vi "Rotation3d_Interpolate.vi"(9 "T":dbl, 10 "EndValue Rotation3d":T1={"Q_quaternion"={"R"=1.0, "V"=[0.0, 0.0, 0.0]}}, 11 "in Rotation3d":T1={"Q_quaternion"={"R"=1.0, "V"=[0.0, 0.0, 0.0]}}) -> (3 "Interpolated Rotation3d":T1={"Q_quaternion"={"R"=1.0, "V"=[0.0, 0.0, 0.0]}})   [LabVIEW 2019, in "Trajectory_Library.lvlib"]
doc: "Interpolates between 2 Rotation3d.\n\nParameters:\n - IN ROTATION3D -- This rotation3d data structure\n - End Value ROTATION3D -- The end rotation3d\n - T -- Interpolation value between 0 and 1.\n\nReturns:\n- Interpolated Rotation3d -- The Rotation3d interpolated betwee the 2 provided interpolations."
uses:
  Trajectory_Library.lvlib
  ROTATION3D.ctl
  QUATERNION.ctl
  Rotation3d_UnaryMinus.vi
  Rotation3d_RotateBy.vi
  Rotation3d_Create_AxisAngle.vi
  Rotation3d_GetQuaterion.vi
  Quaternion_Get_Vect.vi
  Quaternion_Get_W.vi
  Rotation3d_Create_Quaternion.vi
  Quaternion_Inverse.vi
  Quaternion_Times.vi
  Matrix_NormF.vi
  Quaternion_New.vi
  Rotation3d_Create_Default.vi
  Quaternion_Normalize.vi
  <vilib>/Analysis/_algsub.llb/Matrix Norm.vi
  <vilib>/Analysis/_algsub.llb/Real Matrix Norm.vi
  Quaternion_New_Default.vi
  <vilib>/Analysis/Matrix/Numeric/Conversions/Array To Matrix.vi
  <vilib>/Analysis/Matrix/Numeric/Conversions/Array To Matrix - RA.vi
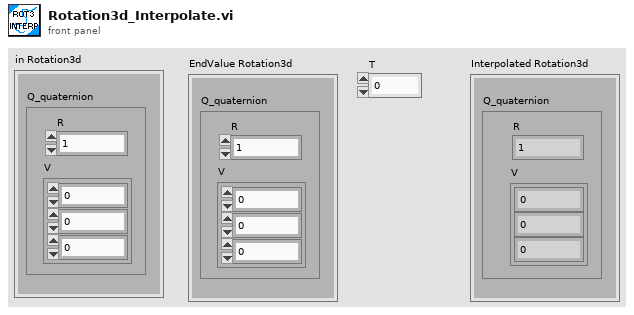
[diagram p1: front panel]
types:
  T1 = typedef "Trajectory_Library.lvlib/ROTATION3D.ctl" = cluster{"Q_quaternion":T2}
  T2 = typedef "Trajectory_Library.lvlib/QUATERNION.ctl" = cluster{"R":dbl, "V":dbl[]}
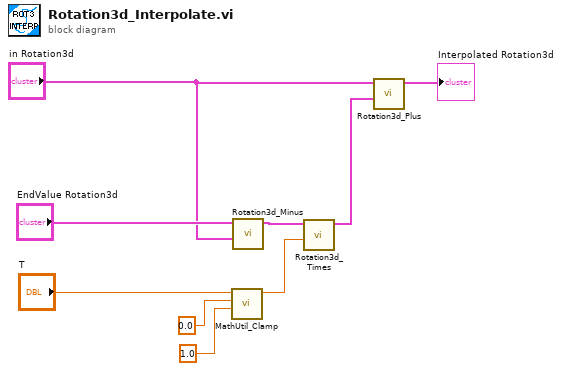
[diagram p0: block diagram]
diagram:
  n1 = call "MathUtil_Clamp.vi"("High Limit"=1.0, "Low Limit"=0.0, "Value"="T") -> ("Result"=w4:dbl)  [unwired: 8 in]
  n2 = call "Rotation3d_Minus.vi"("other Rotation3d"="in Rotation3d", "in Rotation3d"="EndValue Rotation3d") -> ("out Rotation3d"=w8:T1)  [unwired: 9 in]
  n3 = call "Rotation3d_Times.vi"("Scalar"=w4, "in Rotation3d"=w8) -> ("out Rotation3d"=w1:T1)  [unwired: 9 in]
  n4 = call "Rotation3d_Plus.vi"("other Rotation3d"=w1, "in Rotation3d"="in Rotation3d") -> ("out Rotation3d"=→"Interpolated Rotation3d":T1)  [unwired: 9 in]
